vi "PH_BeamlineController.Path set Target.vi"(0 "i ref in":refnum<vi>, 5 "error in (no error)":errorcluster) -> (14 "i ref out":refnum<vi>, 17 "Path changed?":bool, 19 "error out":errorcluster)   [LabVIEW 2014, in "PH_BeamlineController.lvlib"]
doc: "This VI writes incoming Information to own Attributes if the new value differs from the stored."
uses:
  PH_BeamlineController.lvlib
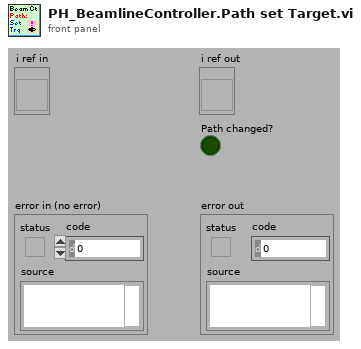
[diagram p1: front panel]
types:
  T1 = typedef "PH_BeamlineController.lvlib/PH_BeamlineController.Target Attributes.ctl" = cluster{"Name":T2, "GUI Ref":refnum<vi>, "Current State":bool, "Wanted State":bool, "Enabled":bool}
  T2 = typedef "PH_BeamlineController.lvlib/PH_BeamlineController.Targets.ctl" = enum16{"None", "PreAmp", "Dump Exp Laserlab", "Exp Laserlab", "Calorimeter", "Dump Exp Laserbay", "Exp Laserbay", "Dump Exp Z6", "Exp Z6"}
  T3 = typedef "PH_BeamlineController.lvlib/PH_BeamlineController.i attribute.ctl" = cluster{"Vacuum Exp LB":cluster{"Channel":string, "Limit [mbar]":dbl, "Pressure [mbar]":dbl, "GUI Ref":refnum<vi>}, "Sources":T4[], "PA DP Targets":T6[], "Path":cluster{"Source":T5, "PA DP Target":T7, "Target":T2}, "Targets":cluster{"Name":T2, "GUI Ref":refnum<vi>, "Current State":bool, "Wanted State":bool, "Enabled":bool}[], "Status Tags":cluster{"Name":string, "Status":T8}[], "special GUI Refs":T9}
  T4 = typedef "PH_BeamlineController.lvlib/PH_BeamlineController.Source Attributes.ctl" = cluster{"Name":T5, "GUI Ref":refnum<vi>, "Current State":bool, "Wanted State":bool}
  T5 = typedef "PH_BeamlineController.lvlib/PH_BeamlineController.Sources.ctl" = enum16{"None", "YLF", "fs-Frontend", "ns-Frontend", "YLF and ns-Frontend", "fs- and ns-Frontend"}
  T6 = typedef "PH_BeamlineController.lvlib/PH_BeamlineController.PA DP Target Attributes.ctl" = cluster{"Name":T7, "GUI Ref":refnum<vi>, "Current State":bool, "Wanted State":bool, "Enabled":bool}
  T7 = typedef "PH_BeamlineController.lvlib/PH_BeamlineController.PA DP Targets.ctl" = enum16{"None", "Dump PA Delayed Beam", "Dump PA Undelayed Beam", "Dumps PA Delayed and Undelayed Beam"}
  T8 = typedef "PH_StatusHandler.lvlib/PH_StatusHandler.Status.ctl" = i16
  T9 = typedef "PH_BeamlineController.lvlib/PH_BeamlineController.special GUI Refs.ctl" = cluster{"PA-Backreflection-Meas":refnum<vi>, "fs_Synchrolock_Watch":refnum<vi>}
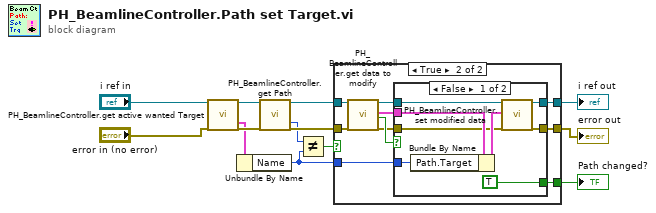
[diagram p0: block diagram]
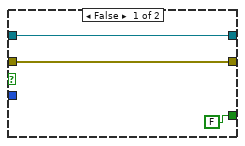
[diagram p2: hidden frame]
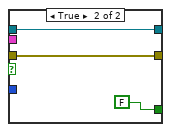
[diagram p3: hidden frame]
diagram:
  n1 = call "PH_BeamlineController.get active wanted Target.vi"("VI in"="i ref in", "error in (no error)"="error in (no error)") -> ("VI out"=w3:refnum<vi>, "active wanted State Target Attributes"=w2:T1, "error out"=w7:errorcluster)  [unwired: 14 in, 1 out]
  n2 = Unbundle By Name(w2) -> ("Name"=w1:T2)
  n3 = call "PH_BeamlineController.get Path.vi"("VI in"=w3, "error in (no error)"=w7) -> ("VI out"=w9:refnum<vi>, "Path: Target"=w4:T2, "error out"=w8:errorcluster)  [unwired: 12 in, 3 out]
  n4 = Not Equal?(x=w4, y=w1) -> (x != y?=w10:bool)
  n5 = case shown="True" w10 {
    tunnel: w1 -> [_ w26]
    tunnel: [w16 w21] -> w12
    tunnel: [w15 w20] -> w13
    tunnel: w8 -> [w15 w19]
    tunnel: w9 -> [w16 w18]
    tunnel: [FALSE w17] -> w11
    frame False {
    }
    frame True {
      n6 = call "PH_BeamlineController.get data to modify.vi"("i ref in"=w18, "error in (no error)"=w19) -> ("i ref out"=w22:refnum<vi>, "i attribute"=w24:T3, "timed out"=w25:bool, "error out"=w23:errorcluster)  [unwired: 14 in]
      n7 = case shown="False" w25 {
        tunnel: w22 -> [w30 w37]
        tunnel: [w34 w37] -> w21
        tunnel: w23 -> [w29 w36]
        tunnel: [w33 w36] -> w20
        tunnel: w24 -> [w32 _]
        tunnel: w26 -> [w27 _]
        tunnel: [TRUE FALSE] -> w17
        frame False {
          n8 = Bundle By Name(cluster=w32, "Path.Target"=w27) -> (w31:T3)
          n9 = call "PH_BeamlineController.set modified data.vi"("i ref in"=w30, "i attribute"=w31, "error in (no error)"=w29) -> ("i ref out"=w34:refnum<vi>, "error out"=w33:errorcluster)  [unwired: 15 in]
        }
        frame True {
        }
      }
    }
  }
  "error out" <- w13
  "i ref out" <- w12
  "Path changed?" <- w11
